vi "13Sheridan.vi"() -> ()   [LabVIEW 2014]
panel:
  out "Temperature Graph":dbl[](graph)
  out "Threshold Status":bool
  out "Indicator":dbl[](array[numeric])
  in  "Control":dbl[](array[numeric])
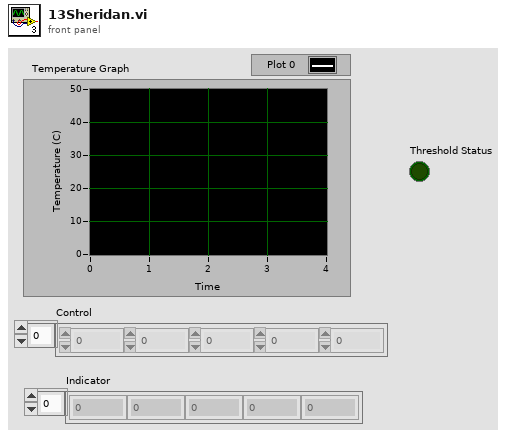
[diagram p1: front panel]
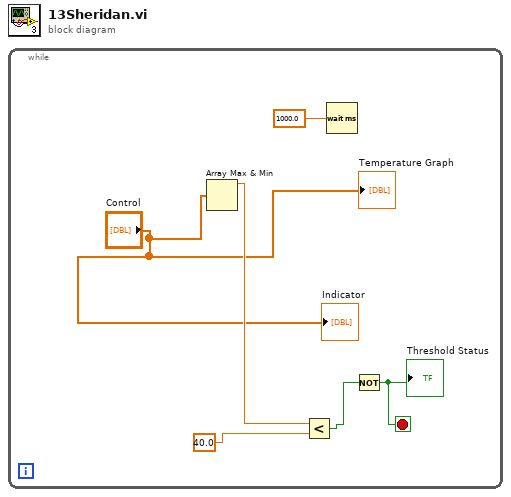
[diagram p0: block diagram]
diagram:
  n1 = while {
    stop <- w1 stop-if-true
    n2 = Array Max & Min(array="Control") -> (max value=w5:dbl)  [unwired: 3 out]
    n3 = Less?(x=w5, y=40.0) -> (x < y?=w2:bool)
    n4 = Wait (ms)(milliseconds to wait=1000.0) -> ()  [unwired: 1 out]
    n5 = Not(x=w2) -> (.not. x?=w1:bool)
    "Threshold Status" <- w1
    "Indicator" <- "Control"
    "Temperature Graph" <- "Control"
  }
